vi "Three part tester simplified.vi"() -> ()   [LabVIEW 2009]
uses:
  <vilib>/Instr/_visa.llb/VISA Configure Serial Port (Instr).vi
panel:
  out "Cluster Display":T1
  in  "Stop":bool
  out "decimal integer string 2":string
  out "number 2":u8 format="%b"
  in  "Orange Bass LED":bool
  in  "Yellow Bass LED":bool
  in  "Green Bass LED":bool
  in  "Red Bass LED":bool
  in  "Blue Bass LED":bool
  in  "Red Drum":bool
  in  "VISA resource name":refnum<visa-resource-name>
  in  "Yellow Drum":bool
  # "Drums"
  # "Bass"
  # "Guitar"
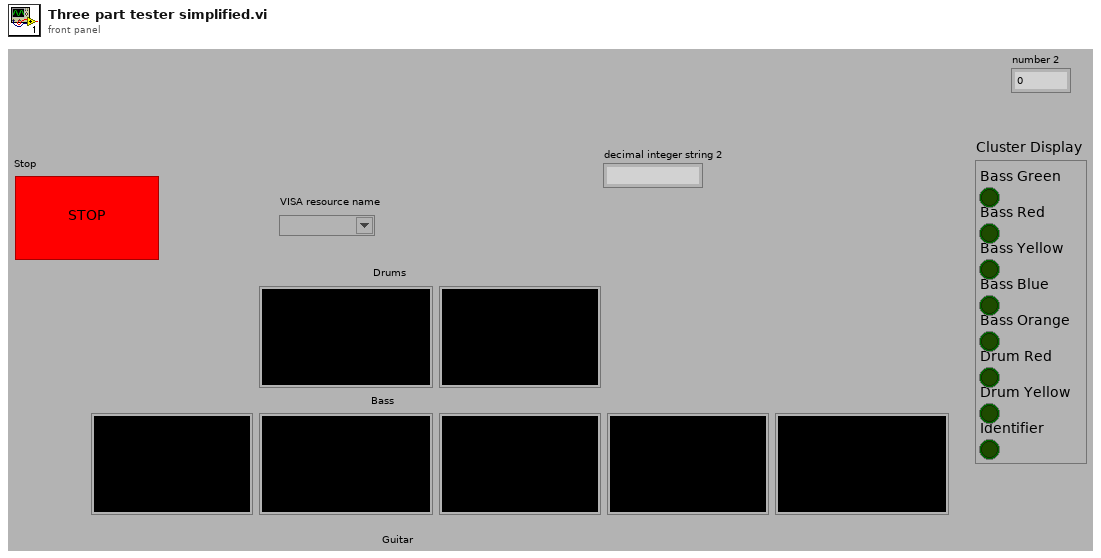
[diagram p1: front panel]
types:
  T1 = cluster{"Bass Green":bool, "Bass Red":bool, "Bass Yellow":bool, "Bass Blue":bool, "Bass Orange":bool, "Drum Red":bool, "Drum Yellow ":bool, "Identifier":bool}
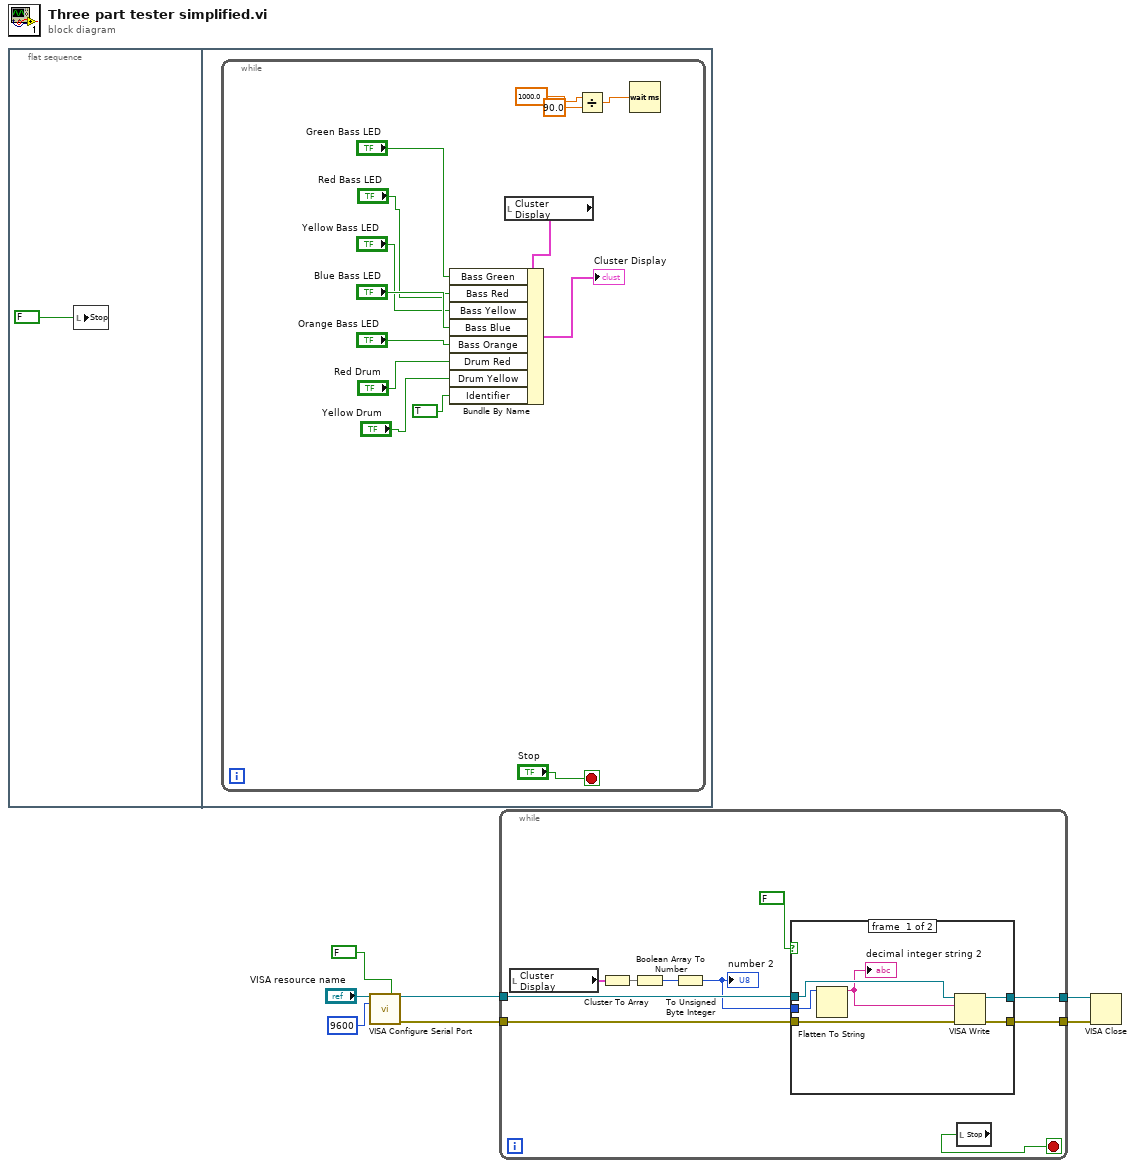
[diagram p0: block diagram]
diagram:
  n1 = flat-sequence {
    frame #0 {
      n2 = local write "Stop"(FALSE ("Stop 2")) -> ()
    }
    frame #1 {
      n3 = while {
        stop <- "Stop" stop-if-true
        n4 = local read "Cluster Display"() -> (w21:T1)
        n5 = Bundle By Name(cluster=w21, "Bass Green"="Green Bass LED", "Bass Red"="Red Bass LED", "Bass Yellow"="Yellow Bass LED", "Bass Blue"="Blue Bass LED", "Bass Orange"="Orange Bass LED", "Drum Red"="Red Drum", "Drum Yellow"="Yellow Drum", "Identifier"=TRUE ("element")) -> (→"Cluster Display":T1)
        n6 = Divide(x=1000.0, y=90.0) -> (x/y=w9:dbl)
        n7 = Wait (ms)(milliseconds to wait=w9) -> ()  [unwired: 1 out]
      }
    }
  }
  n8 = call-poly "VISA Configure Serial Port"("VISA resource name"="VISA resource name", "Enable Termination\nChar (T)"=FALSE ("Enable Termination\nChar (T)"), "baud rate (9600)"=u32 9600) -> ("VISA resource name out"=w7:refnum<visa-resource-name>, "error out"=w2:errorcluster)  [unwired: 11 in]
  n9 = while {
    tunnel: w7 -> [w32]
    tunnel: [w31] -> w6
    tunnel: w2 -> [w30]
    tunnel: [w29] -> w1
    stop <- w26 stop-if-true
    n10 = local read "Cluster Display"() -> (w27:T1)
    n11 = Cluster To Array(cluster=w27) -> (array=w28:bool[])
    n12 = Boolean Array To Number(Boolean array=w28) -> (number=w24:u32)
    n13 = To Unsigned Byte Integer(number=w24) -> (unsigned 8bit integer=w23:u8)
    "number 2" <- w23
    n14 = case shown="False" FALSE ("Send") {
      tunnel: w32 -> [w38 w40]
      tunnel: [w37 w40] -> w31
      tunnel: w30 -> [w36 w39]
      tunnel: [w35 w39] -> w29
      tunnel: w23 -> [w34 _]
      frame #0 {
        n15 = Flatten To String(anything=w34) -> (data string=w33:string)  [unwired: 3 in, 2 out]
        "decimal integer string 2" <- w33
        n16 = VISA Write(VISA resource name=w38, write buffer=w33, error in (no error)=w36) -> (VISA resource name out=w37:refnum<visa-resource-name>, error out=w35:errorcluster)  [unwired: 1 out]
      }
      frame #1 {
      }
    }
    n17 = local read "Stop"() -> (w26:bool)
  }
  n18 = VISA Close(VISA resource name=w6, error in (no error)=w1) -> ()  [unwired: 1 out]
